vi "Get XML Attributes.vi"(8 "error in (no error)":errorcluster, 11 "Element in":refnum<class "Element.lvclass">) -> (0 "error out":errorcluster, 2 "XML Attributes":cluster{"Name":string, "Value":string}[](array[cluster]), 3 "Element out":refnum<class "Element.lvclass">)   [LabVIEW 2023, in "VILab.lvlib" / "Element.lvclass"]
uses:
  Element.lvclass
  Element.lvclass/Element.ctl
  Data Item.lvclass
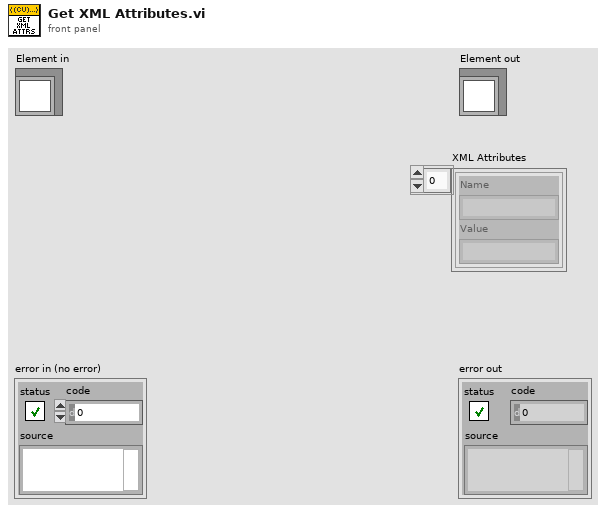
[diagram p1: front panel]
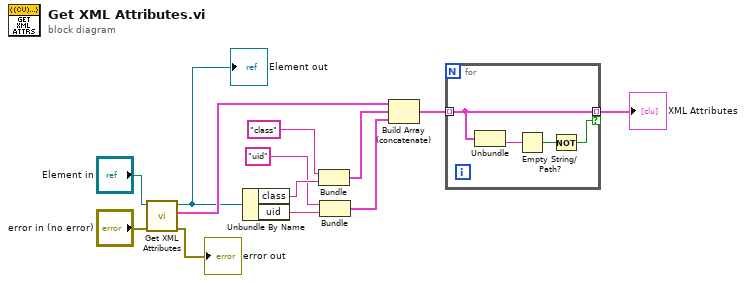
[diagram p0: block diagram]
diagram:
  n1 = call-parent "Get XML Attributes.vi"("error in (no error)"="error in (no error)", "Data Item in"="Element in") -> ("error out"=→"error out":errorcluster, "XML Attributes"=w7:cluster{"Name":string, "Value":string}[], "Data Item out"=w4:refnum<class "Element.lvclass">)  [unwired: 7 in]
  "Element out" <- w4
  n2 = Unbundle By Name(w4) -> ("class"=w11:string, "uid"=w10:string)
  n3 = Bundle("class", "class"=w11) -> (w6:cluster{string, "class":string})  [unwired: 1 in]
  n4 = Bundle("uid", "uid"=w10) -> (w5:cluster{string, "uid":string})  [unwired: 1 in]
  n5 = Build Array (concatenate)(w7, w6, w5) -> (w2:cluster{"Name":string, "uid":string}[])
  n6 = for {
    tunnel: w2 -> [w15] mode=indexing
    tunnel: [w15] -> w1 mode=indexing if=w14
    n7 = Unbundle(w15) -> ("uid"=w17:string)  [unwired: 1 out]
    n8 = Empty String/Path?(string/path=w17) -> (empty?=w16:bool)
    n9 = Not(x=w16) -> (.not. x?=w14:bool)
  }
  "XML Attributes" <- w1
